vi "Build_Installer.vi"(7 "text":string, 8 "error in (no error)":errorcluster, 9 "Build Specification Version":T1, 10 "Workspace path":path, 11 "String in":refnum<vi>) -> (0 "error out":errorcluster)   [LabVIEW 2017]
uses:
  <vilib>/AppBuilder/AB_API_Simple/Build Specification Version.ctl
  BuildItem.ctl
  <vilib>/AppBuilder/AB_API_Simple/NI_App_Builder_API.lvlib
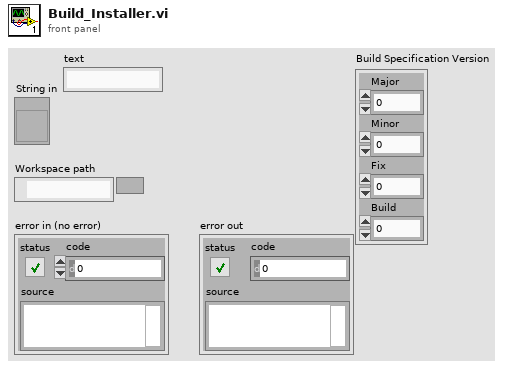
[diagram p1: front panel]
types:
  T1 = typedef "NI_App_Builder_API.lvlib/Build Specification Version.ctl" = cluster{"Major":u16, "Minor":u16, "Fix":u16, "Build":u16}
  T2 = typedef "BuildItem.ctl" = cluster{"Project":path, "BuildSpecification":path, "Destination":path}
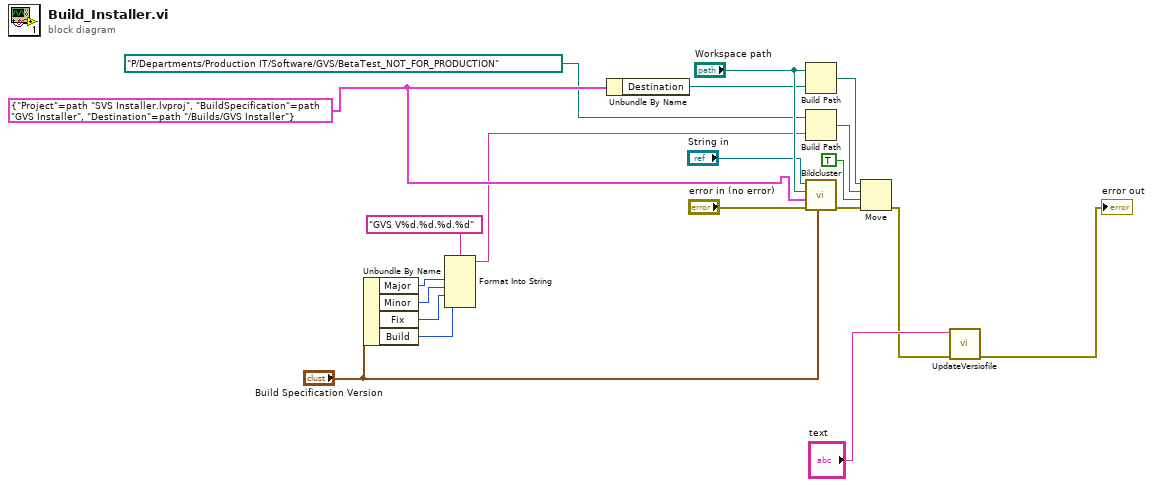
[diagram p0: block diagram]
diagram:
  w13 = T2 {"Project"=path "SVS Installer.lvproj", "BuildSpecification"=path "GVS Installer", "Destination"=path "../Builds/GVS Installer"} ("BuildItem")
  n1 = Unbundle By Name("Build Specification Version") -> ("Major"=w10:u16, "Minor"=w9:u16, "Fix"=w8:u16, "Build"=w7:u16)
  n2 = Format Into String(format string="GVS V%d.%d.%d.%d", w10, w9, w8, w7) -> (resulting string=w1:string)  [unwired: 2 in, 1 out]
  n3 = Unbundle By Name(w13) -> ("Destination"=w18:path)
  n4 = Build Path(base path="Workspace path", name or relative path=w18) -> (appended path=w14:path)
  n5 = Build Path(base path=path "P:/Departments/Production IT/Software/GVS/BetaTest_NOT_FOR_PRODUCTION", name or relative path=w1) -> (appended path=w20:path)
  n6 = call "Bildcluster.vi"("Build Specification Version"="Build Specification Version", "error in (no error)"="error in (no error)", "BuildItem"=w13, "path"="Workspace path", "String in"="String in") -> ("error out"=w5:errorcluster)  [unwired: 6 in]
  n7 = Move(source path=w14, error in=w5, 9:TRUE ("overwrite (F)"), 10:w20) -> (error out=w3:errorcluster)  [unwired: 1 in, 2 out]
  n8 = call "UpdateVersiofile.vi"("error in (no error)"=w3, "msg"="text") -> ("error out"=→"error out":errorcluster)  [unwired: 9 in]
